vi "HSL to RGB.vi"(8 "Error In":errorcluster, 9 "Lum":u8, 10 "Sat":u8, 11 "Hue":u8) -> (0 "Error Out":errorcluster, 1 "Blue":u8, 2 "Green":u8, 3 "Red":u8)   [LabVIEW 2012]
doc: "Converts HSL values (0-240) to RGB values (0-255). RGB colorspace is the display colorspace for web and computer monitors. RGB uses Red, Green and Blue components to form a color. This isn't very useful for programmatically changing a color. HSL colorspace uses Hue, Saturation and Lightness components of a color which can be analyzed, extract or modified in a way to change the function of a color. \n\nSee HSLToolsBasicExample.vi for more information in the NI Example Finder."
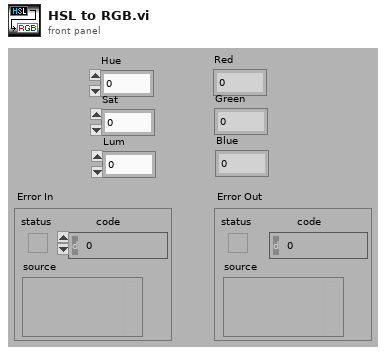
[diagram p1: front panel]
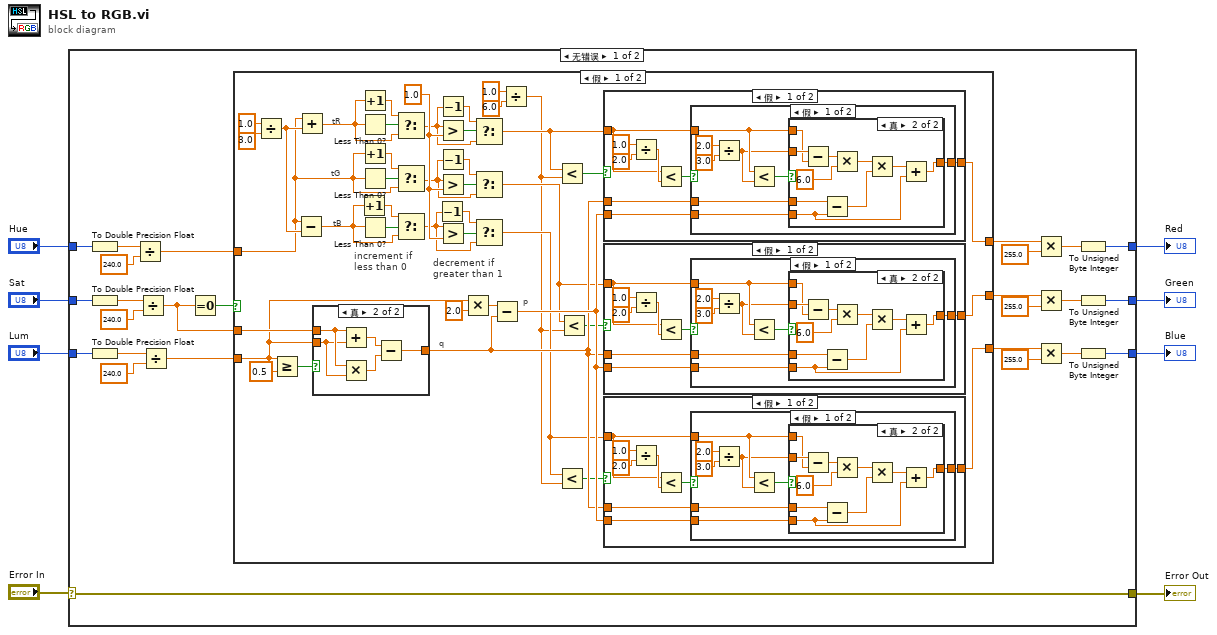
[diagram p0: block diagram]
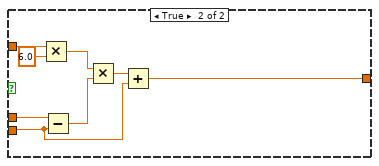
[diagram p4: hidden frame]
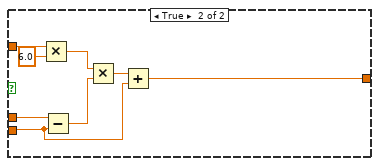
[diagram p7: hidden frame]
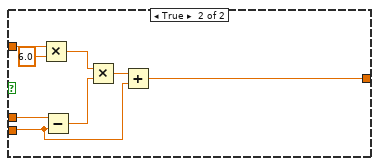
[diagram p10: hidden frame]
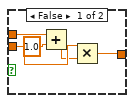
[diagram p11: hidden frame]
diagram:
  n1 = case shown="无错误" "Error In" {
    selector: "Error In" -> [w21 w199]
    tunnel: [w9 w196] -> w8
    tunnel: "Hue" -> [w20 w196]
    tunnel: "Sat" -> [w19 w197]
    tunnel: "Lum" -> [w18 w198]
    tunnel: [w10 w197] -> w4
    tunnel: [w11 w198] -> w3
    tunnel: [w21 w199] -> w1
    frame No Error {
      n2 = To Double Precision Float(number=w20) -> (double precision float=w15:dbl)
      n3 = To Double Precision Float(number=w19) -> (double precision float=w16:dbl)
      n4 = To Double Precision Float(number=w18) -> (double precision float=w17:dbl)
      n5 = Divide(x=w15, y=240.0) -> (x/y=w27:dbl)
      n6 = Divide(x=w16, y=240.0) -> (x/y=w26:dbl)
      n7 = Divide(x=w17, y=240.0) -> (x/y=w25:dbl)
      n8 = Equal To 0?(x=w26) -> (x = 0?=w28:bool)
      n9 = case shown="假" w28 {
        tunnel: w27 -> [w59 _]
        tunnel: w26 -> [w74 _]
        tunnel: w25 -> [w73 w195]
        tunnel: [w37 w195] -> w24
        tunnel: [w36 w195] -> w23
        tunnel: [w35 w195] -> w22
        frame False {
          w52 = 1.0 ("x")
          # "decrement if\ngreater than 1"
          # "increment if\nless than 0"
          # "tB"
          # "tG"
          # "tR"
          # "p"
          # "q"
          n10 = Divide(x=1.0, y=3.0 ("x")) -> (x/y=w68:dbl)
          n11 = Greater Or Equal?(x=w73, y=0.5) -> (x >= y?=w75:bool)
          n12 = Subtract(x=w59, y=w68) -> (x-y=w60:dbl)
          n13 = Add(x=w59, y=w68) -> (x+y=w63:dbl)
          n14 = case shown="真" w75 {
            tunnel: w74 -> [w189 w194]
            tunnel: w73 -> [w187 w193]
            tunnel: [w185 w190] -> w43
            frame False {
              n15 = Add(x=w189, y=1.0) -> (x+y=w186:dbl)
              n16 = Multiply(x=w187, y=w186) -> (x*y=w185:dbl)
            }
            frame True {
              n17 = Add(x=w194, y=w193) -> (x+y=w191:dbl)
              n18 = Multiply(x=w194, y=w193) -> (x*y=w192:dbl)
              n19 = Subtract(x=w191, y=w192) -> (x-y=w190:dbl)
            }
          }
          n20 = Increment(x=w60) -> (x+1=w61:dbl)
          n21 = Increment(x=w63) -> (x+1=w64:dbl)
          n22 = Less Than 0?(x=w63) -> (x < 0?=w66:bool)
          n23 = Increment(x=w59) -> (x+1=w62:dbl)
          n24 = Less Than 0?(x=w59) -> (x < 0?=w67:bool)
          n25 = Less Than 0?(x=w60) -> (x < 0?=w65:bool)
          n26 = Select(t=w64, s=w66, f=w63) -> (s? t:f=w51:dbl)
          n27 = Select(t=w62, s=w67, f=w59) -> (s? t:f=w50:dbl)
          n28 = Select(t=w61, s=w65, f=w60) -> (s? t:f=w49:dbl)
          n29 = Decrement(x=w49) -> (x-1=w58:dbl)
          n30 = Decrement(x=w51) -> (x-1=w56:dbl)
          n31 = Greater?(x=w51, y=w52) -> (0:w54:bool)
          n32 = Decrement(x=w50) -> (x-1=w57:dbl)
          n33 = Greater?(x=w50, y=w52) -> (0:w53:bool)
          n34 = Greater?(x=w49, y=w52) -> (0:w55:bool)
          n35 = Multiply(x=w73, y=2.0) -> (x*y=w71:dbl)
          n36 = Select(t=w56, s=w54, f=w51) -> (s? t:f=w45:dbl)
          n37 = Select(t=w57, s=w53, f=w50) -> (s? t:f=w39:dbl)
          n38 = Select(t=w58, s=w55, f=w49) -> (s? t:f=w40:dbl)
          n39 = Subtract(x=w71, y=w43) -> (x-y=w44:dbl)
          n40 = Divide(x=1.0, y=6.0 ("x")) -> (x/y=w38:dbl)
          n41 = Less?(x=w45, y=w38) -> (x < y?=w48:bool)
          n42 = Less?(x=w40, y=w38) -> (x < y?=w41:bool)
          n43 = Less?(x=w39, y=w38) -> (x < y?=w42:bool)
          n44 = case shown="假" w48 {
            tunnel: w45 -> [w150 w184]
            tunnel: w44 -> [w149 w178]
            tunnel: w43 -> [w152 w182]
            tunnel: [w151 w177] -> w37
            frame False {
              n45 = Divide(x=1.0, y=2.0 ("x")) -> (x/y=w154:dbl)
              n46 = Less?(x=w150, y=w154) -> (x < y?=w153:bool)
              n47 = case shown="假" w153 {
                tunnel: w152 -> [w159 w176]
                tunnel: [w157 w176] -> w151
                tunnel: w150 -> [w161 _]
                tunnel: w149 -> [w158 _]
                frame False {
                  n48 = Divide(x=2.0, y=3.0 ("x")) -> (x/y=w160:dbl)
                  n49 = Less?(x=w161, y=w160) -> (x < y?=w162:bool)
                  n50 = case shown="真" w162 {
                    tunnel: w161 -> [_ w174]
                    tunnel: w160 -> [_ w175]
                    tunnel: w159 -> [_ w171]
                    tunnel: w158 -> [w165 w167]
                    tunnel: [w165 w166] -> w157
                    frame False {
                    }
                    frame True {
                      n51 = Subtract(x=w175, y=w174) -> (x-y=w173:dbl)
                      n52 = Subtract(x=w171, y=w167) -> (x-y=w169:dbl)
                      n53 = Multiply(x=w173, y=6.0) -> (x*y=w170:dbl)
                      n54 = Multiply(x=w170, y=w169) -> (x*y=w168:dbl)
                      n55 = Add(x=w168, y=w167) -> (x+y=w166:dbl)
                    }
                  }
                }
                frame True {
                }
              }
            }
            frame True {
              n56 = Multiply(x=w184, y=6.0) -> (x*y=w181:dbl)
              n57 = Subtract(x=w182, y=w178) -> (x-y=w180:dbl)
              n58 = Multiply(x=w181, y=w180) -> (x*y=w179:dbl)
              n59 = Add(x=w179, y=w178) -> (x+y=w177:dbl)
            }
          }
          n60 = case shown="假" w42 {
            tunnel: w39 -> [w114 w148]
            tunnel: w44 -> [w113 w142]
            tunnel: w43 -> [w116 w146]
            tunnel: [w115 w141] -> w36
            frame False {
              n61 = Divide(x=1.0, y=2.0 ("x")) -> (x/y=w118:dbl)
              n62 = Less?(x=w114, y=w118) -> (x < y?=w117:bool)
              n63 = case shown="假" w117 {
                tunnel: w116 -> [w123 w140]
                tunnel: [w121 w140] -> w115
                tunnel: w114 -> [w125 _]
                tunnel: w113 -> [w122 _]
                frame False {
                  n64 = Divide(x=2.0, y=3.0 ("x")) -> (x/y=w124:dbl)
                  n65 = Less?(x=w125, y=w124) -> (x < y?=w126:bool)
                  n66 = case shown="真" w126 {
                    tunnel: w125 -> [_ w138]
                    tunnel: w124 -> [_ w139]
                    tunnel: w123 -> [_ w135]
                    tunnel: w122 -> [w129 w131]
                    tunnel: [w129 w130] -> w121
                    frame False {
                    }
                    frame True {
                      n67 = Subtract(x=w139, y=w138) -> (x-y=w137:dbl)
                      n68 = Subtract(x=w135, y=w131) -> (x-y=w133:dbl)
                      n69 = Multiply(x=w137, y=6.0) -> (x*y=w134:dbl)
                      n70 = Multiply(x=w134, y=w133) -> (x*y=w132:dbl)
                      n71 = Add(x=w132, y=w131) -> (x+y=w130:dbl)
                    }
                  }
                }
                frame True {
                }
              }
            }
            frame True {
              n72 = Multiply(x=w148, y=6.0) -> (x*y=w145:dbl)
              n73 = Subtract(x=w146, y=w142) -> (x-y=w144:dbl)
              n74 = Multiply(x=w145, y=w144) -> (x*y=w143:dbl)
              n75 = Add(x=w143, y=w142) -> (x+y=w141:dbl)
            }
          }
          n76 = case shown="假" w41 {
            tunnel: w40 -> [w78 w112]
            tunnel: w44 -> [w77 w106]
            tunnel: w43 -> [w80 w110]
            tunnel: [w79 w105] -> w35
            frame False {
              n77 = Divide(x=1.0, y=2.0 ("x")) -> (x/y=w82:dbl)
              n78 = Less?(x=w78, y=w82) -> (x < y?=w81:bool)
              n79 = case shown="假" w81 {
                tunnel: w80 -> [w87 w104]
                tunnel: [w85 w104] -> w79
                tunnel: w78 -> [w89 _]
                tunnel: w77 -> [w86 _]
                frame False {
                  n80 = Divide(x=2.0, y=3.0 ("x")) -> (x/y=w88:dbl)
                  n81 = Less?(x=w89, y=w88) -> (x < y?=w90:bool)
                  n82 = case shown="真" w90 {
                    tunnel: w89 -> [_ w102]
                    tunnel: w88 -> [_ w103]
                    tunnel: w87 -> [_ w99]
                    tunnel: w86 -> [w93 w95]
                    tunnel: [w93 w94] -> w85
                    frame False {
                    }
                    frame True {
                      n83 = Subtract(x=w103, y=w102) -> (x-y=w101:dbl)
                      n84 = Subtract(x=w99, y=w95) -> (x-y=w97:dbl)
                      n85 = Multiply(x=w101, y=6.0) -> (x*y=w98:dbl)
                      n86 = Multiply(x=w98, y=w97) -> (x*y=w96:dbl)
                      n87 = Add(x=w96, y=w95) -> (x+y=w94:dbl)
                    }
                  }
                }
                frame True {
                }
              }
            }
            frame True {
              n88 = Multiply(x=w112, y=6.0) -> (x*y=w109:dbl)
              n89 = Subtract(x=w110, y=w106) -> (x-y=w108:dbl)
              n90 = Multiply(x=w109, y=w108) -> (x*y=w107:dbl)
              n91 = Add(x=w107, y=w106) -> (x+y=w105:dbl)
            }
          }
        }
        frame True {
        }
      }
      n92 = Multiply(x=w24, y=255.0) -> (x*y=w12:dbl)
      n93 = Multiply(x=w23, y=255.0) -> (x*y=w13:dbl)
      n94 = Multiply(x=w22, y=255.0) -> (x*y=w14:dbl)
      n95 = To Unsigned Byte Integer(number=w12) -> (unsigned 8bit integer=w9:u8)
      n96 = To Unsigned Byte Integer(number=w13) -> (unsigned 8bit integer=w10:u8)
      n97 = To Unsigned Byte Integer(number=w14) -> (unsigned 8bit integer=w11:u8)
    }
    frame Error {
    }
  }
  "Red" <- w8
  "Green" <- w4
  "Blue" <- w3
  "Error Out" <- w1
